vi "FM_RTL-SDR_RX-DLL_X64.vi"() -> ()   [LabVIEW 2013]
uses:
  <vilib>/sound2/lvsound2.llb/Sound Data Format.ctl
  <vilib>/sound2/lvsound2.llb/Sound Output Write (DBL Single).vi
  <vilib>/Analysis/2dsp.llb/Rational Resample (single channel, DBL).vi
  <instrlib>/rtlsdr/rtlsdrx64.lvlib
  <vilib>/Analysis/NI_AALPro.lvlib
  <userlib>/FMDemodRTLSDR_Script/FMDemodRTLSDR_Script.dll
panel:
  out "Boolean":bool
  out "error out":errorcluster
  out "error out":errorcluster
  in  "Device index":u32
  out "Samples Acquired":u32
  out "DevRefnum":u64
  out "error out":errorcluster
  in  "sound format":T1={"sample rate (S/s)"=44100.0, "number of channels"=1, "bits per sample"=16}
  in  "stop":bool
  in  "中心频率：":u32(slide)=104300000 scale=86000000.0..108000000.0 scale format="%#_6p"
  in  "IQ rate":u32=286650
  out "error out":errorcluster
  # "FM Receiver"
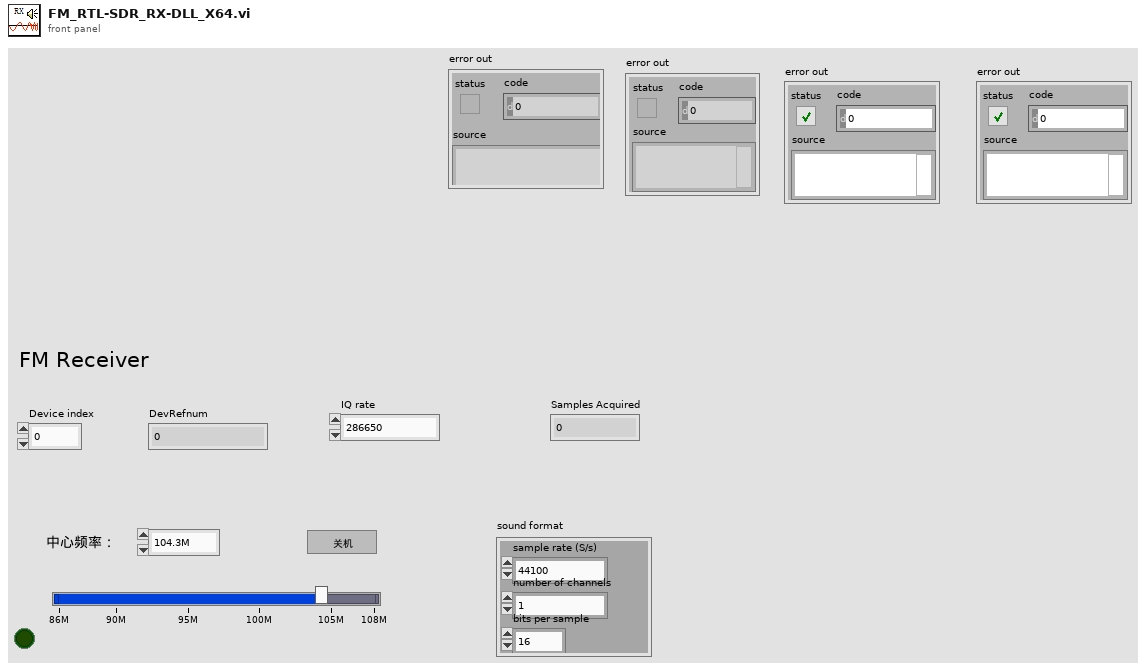
[diagram p1: front panel]
types:
  T1 = typedef "Sound Data Format.ctl" = cluster{"sample rate (S/s)":dbl, "number of channels":i32, "bits per sample":i32}
  T2 = typedef "Sound Output Task ID.ctl" = u32
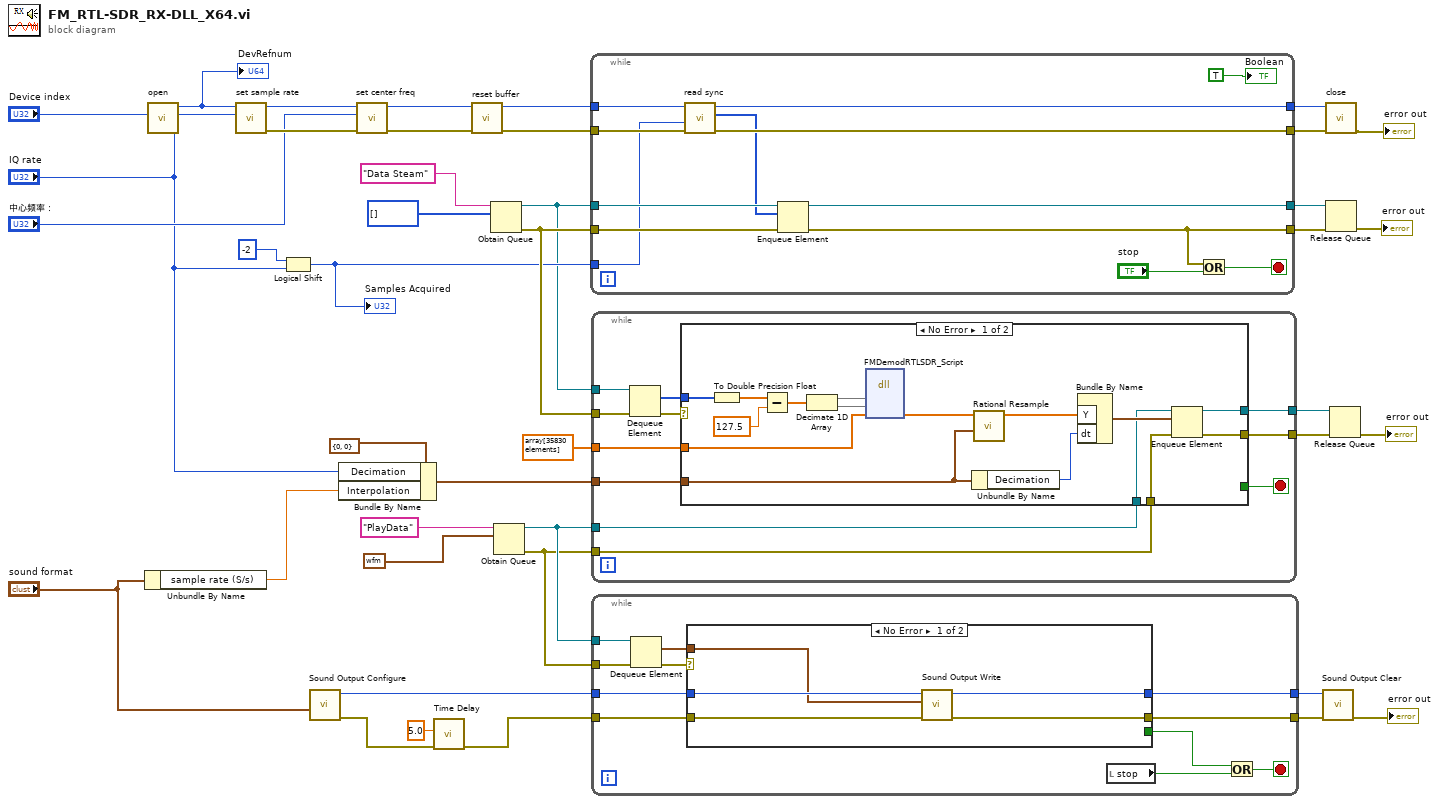
[diagram p0: block diagram]
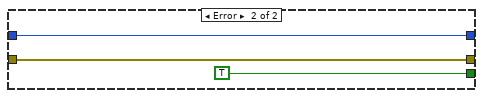
[diagram p2: hidden frame]
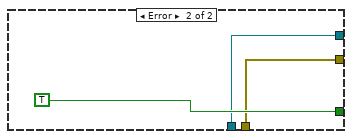
[diagram p3: hidden frame]
diagram:
  n1 = Unbundle By Name("sound format") -> ("sample rate (S/s)"=w14:dbl)
  n2 = call <instrlib>:"open.vi"("index"="Device index") -> ("DevRefnum"=w34:u64)  [unwired: 9 in, 1 out]
  "DevRefnum" <- w34
  n3 = call <instrlib>:"set sample rate.vi"("rate"="IQ rate", "DevRefnum"=w34) -> ("error out"=w36:errorcluster, "DevRefnum"=w38:u64)  [unwired: 7 in, 1 out]
  n4 = Logical Shift(y=i16 -2, x="IQ rate") -> (x << y=w17:u32)
  "Samples Acquired" <- w17
  n5 = call <vilib>:"Sound Output Configure.vi"("sound format"="sound format") -> ("error out"=w21:errorcluster, "task ID"=w10:T2)  [unwired: 9 in]
  n6 = Bundle By Name(cluster=cluster{"Interpolation":i32, "Decimation":i32} {"Interpolation"=0, "Decimation"=0}, "Decimation"="IQ rate", "Interpolation"=w14) -> (w22:cluster{"Interpolation":i32, "Decimation":i32})
  n7 = call <instrlib>:"set center freq.vi"("error in (no error)"=w36, "freq"="中心频率：", "DevRefnum"=w38) -> ("error out"=w35:errorcluster, "DevRefnum"=w37:u64)  [unwired: 6 in, 1 out]
  n8 = call "Time Delay"("error in (no error)"=w21, "Delay Time (s)"=5.0) -> ("error out"=w7:errorcluster)  [unwired: 9 in]
  n9 = call <instrlib>:"reset buffer.vi"("error in (no error)"=w35, "DevRefnum"=w37) -> ("error out"=w31:errorcluster, "DevRefnum"=w32:u64)  [unwired: 8 in]
  n10 = Obtain Queue(name (unnamed)="Data Steam", element data type=u8[] [] ("buf 2")) -> (queue out=w16:refnum<queue>, error out=w18:errorcluster)  [unwired: 3 in, 1 out]
  n11 = Obtain Queue(name (unnamed)="PlayData", element data type=waveform(dbl) {"t0"=timestamp(0 s since 1904-01-01), "dt"=1.0, "Y"=[]} ("waveform")) -> (queue out=w8:refnum<queue>, error out=w4:errorcluster)  [unwired: 3 in, 1 out]
  n12 = while {
    tunnel: [w52] -> w29
    tunnel: w32 -> [w54]
    tunnel: w31 -> [w53]
    tunnel: [w51] -> w28
    tunnel: w17 -> [w43]
    tunnel: w16 -> [w50]
    tunnel: [w49] -> w25
    tunnel: w18 -> [w48]
    tunnel: [w46] -> w24
    stop <- w44 stop-if-true
    n13 = call <instrlib>:"read sync.vi"("error in (no error)"=w53, "len"=w43, "DevRefnum"=w54) -> ("error out"=w51:errorcluster, "buf 2"=w47:u8[], "DevRefnum"=w52:u64)  [unwired: 6 in]
    n14 = Enqueue Element(queue=w50, element=w47, error in (no error)=w48) -> (queue out=w49:refnum<queue>, error out=w46:errorcluster)  [unwired: 1 in, 1 out]
    n15 = Or(x=w46, y="stop") -> (x .or. y?=w44:bool)
    "Boolean" <- TRUE
  }
  n16 = while {
    tunnel: w16 -> [w65]
    tunnel: w22 -> [w59]
    tunnel: w18 -> [w63]
    tunnel: dbl[] array[35830 elements] ("Phase_Diff") -> [w61]
    tunnel: w8 -> [w58]
    tunnel: w4 -> [w57]
    tunnel: [w56] -> w2
    tunnel: [w55] -> w1
    stop <- w60 stop-if-true
    n17 = Dequeue Element(queue=w65, error in (no error)=w63) -> (element=w64:u8[], error out=w62:errorcluster)  [unwired: 1 in, 2 out]
    n18 = case shown="No Error" w62 {
      tunnel: w64 -> [w78 _]
      tunnel: w61 -> [w75 _]
      tunnel: [_ TRUE] -> w60
      tunnel: w59 -> [w72 _]
      tunnel: w58 -> [w70 w83]
      tunnel: w57 -> [w69 w82]
      tunnel: [w68 w83] -> w56
      tunnel: [w67 w82] -> w55
      frame No Error {
        n19 = To Double Precision Float(number=w78) -> (double precision float=w81:dbl[])
        n20 = Subtract(x=w81, y=127.5) -> (x-y=w79:dbl[])
        n21 = Decimate 1D Array(w79) -> (w77:dbl[], w76:dbl[])
        n22 = dll-call lib="C:/Program Files/National Instruments/LabVIEW 2013/user.lib/FMDemodRTLSDR_Script/FMDemodRTLSDR_Script.*" fn="FMDemodRTLSDR_Script"("ISamples"=w77, "QSamples"=w76, "Phase_Diff"=w75) -> ("Phase_Diff"=w66:dbl[])  [unwired: 6 in, 2 out]
        n23 = Unbundle By Name(w72) -> ("Decimation"=w73:i32)
        n24 = call-poly <vilib>:"Rational Resample.vi"("resample factor"=w72, "X"=w66) -> ("Y"=w74:dbl[])  [unwired: 7 in, 2 out]
        n25 = Bundle By Name ("Build Waveform")("Y"=w74, "dt"=w73) -> (w71:waveform(dbl))  [unwired: 1 in]
        n26 = Enqueue Element(queue=w70, element=w71, error in (no error)=w69) -> (queue out=w68:refnum<queue>, error out=w67:errorcluster)  [unwired: 1 in, 1 out]
      }
      frame Error {
      }
    }
  }
  n27 = while {
    tunnel: w10 -> [w95]
    tunnel: [w94] -> w9
    tunnel: w8 -> [w93]
    tunnel: w4 -> [w92]
    tunnel: w7 -> [w91]
    tunnel: [w90] -> w6
    stop <- w85 stop-if-true
    n28 = Dequeue Element(queue=w93, error in (no error)=w92) -> (element=w88:waveform(dbl), error out=w89:errorcluster)  [unwired: 1 in, 2 out]
    n29 = case shown="No Error" w89 {
      tunnel: w95 -> [w100 w103]
      tunnel: [w99 w103] -> w94
      tunnel: w91 -> [w98 w102]
      tunnel: [w97 w102] -> w90
      tunnel: w88 -> [w96 _]
      tunnel: [_ TRUE] -> w87
      frame No Error {
        n30 = call-poly <vilib>:"Sound Output Write.vi"("error in (no error)"=w98, "data"=w96, "task ID"=w100) -> ("error out"=w97:errorcluster, "task ID out"=w99:T2)  [unwired: 7 in]
      }
      frame Error {
      }
    }
    n31 = local read "stop"() -> (w86:bool)
    n32 = Or(x=w87, y=w86) -> (x .or. y?=w85:bool)
  }
  n33 = call <vilib>:"Sound Output Clear.vi"("error in (no error)"=w6, "task ID"=w9) -> ("error out"=→"error out":errorcluster)  [unwired: 9 in]
  n34 = call <instrlib>:"close.vi"("error in (no error)"=w28, "DevRefnum"=w29) -> ("error out"=→"error out":errorcluster)  [unwired: 8 in, 1 out]
  n35 = Release Queue(queue=w25, error in (no error)=w24) -> (error out=→"error out":errorcluster)  [unwired: 1 in, 2 out]
  n36 = Release Queue(queue=w2, error in (no error)=w1) -> (error out=→"error out":errorcluster)  [unwired: 1 in, 2 out]
